vi "HW_Setup.vi"(0 "VISA resource name in":refnum<visa-resource-name>="ASRL3::INSTR", 1 "Traget FPS":i32=80, 2 "Close port? (T)":bool=TRUE, 3 "error in":errorcluster) -> (5 "Version information":string, 6 "VISA resource name out":refnum<visa-resource-name>="ASRL3::INSTR", 7 "Data flow controls":T1, 8 "Instrument OK?":bool=TRUE, 9 "error out":errorcluster)   [LabVIEW 2016]
panel:
  out "FPS status":i32=80
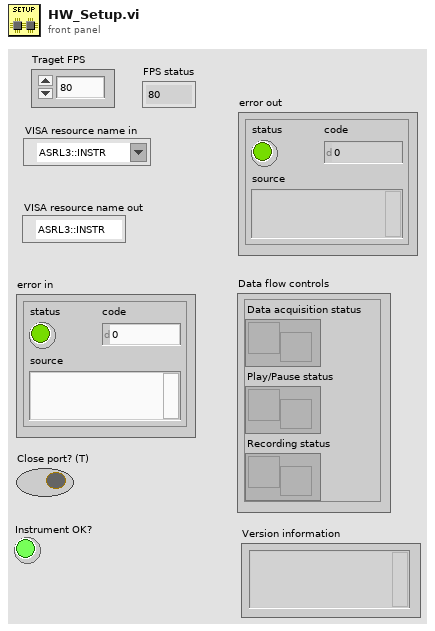
[diagram p1: front panel]
types:
  T1 = cluster{"Data acquisition status":refnum<notifier>, "Play/Pause status":refnum<notifier>, "Recording status":refnum<notifier>}
  T2 = cluster{"notifier out":refnum<notifier>, "notifier out":refnum<notifier>, "notifier out":refnum<notifier>}
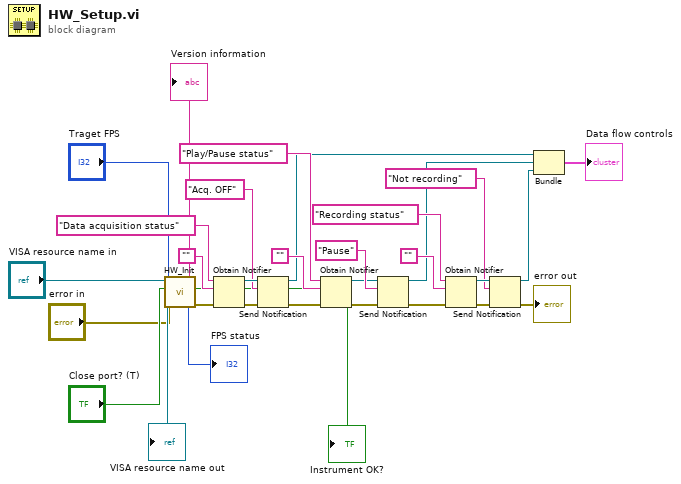
[diagram p0: block diagram]
diagram:
  n1 = call "HW_Init.vi"("error in"="error in", "Traget FPS"="Traget FPS", "Close port? (T)"="Close port? (T)", "VISA resource name"="VISA resource name in") -> ("error out"=w29:errorcluster, "Instrument OK?"=→"Instrument OK?":bool, "VISA resource name out"=→"VISA resource name out":refnum<visa-resource-name>, "FPS status"=→"FPS status":i32, "Version information"=→"Version information":string)  [unwired: 1 out]
  n2 = Obtain Notifier(name (unnamed)="Data acquisition status", notification data type="", error in (no error)=w29) -> (notifier out=w26:refnum<notifier>, error out=w24:errorcluster)  [unwired: 1 in, 1 out]
  n3 = Send Notification(notification="Acq. OFF", notifier=w26, error in (no error)=w24) -> (notifier out=w10:refnum<notifier>, error out=w18:errorcluster)
  n4 = Obtain Notifier(name (unnamed)="Play/Pause status", notification data type="", error in (no error)=w18) -> (notifier out=w21:refnum<notifier>, error out=w23:errorcluster)  [unwired: 1 in, 1 out]
  n5 = Send Notification(notification="Pause", notifier=w21, error in (no error)=w23) -> (notifier out=w9:refnum<notifier>, error out=w12:errorcluster)
  n6 = Obtain Notifier(name (unnamed)="Recording status", notification data type="", error in (no error)=w12) -> (notifier out=w15:refnum<notifier>, error out=w13:errorcluster)  [unwired: 1 in, 1 out]
  n7 = Send Notification(notification="Not recording", notifier=w15, error in (no error)=w13) -> (notifier out=w8:refnum<notifier>, error out=→"error out":errorcluster)
  n8 = Bundle("notifier out"=w10, "notifier out"=w9, "notifier out"=w8) -> (→"Data flow controls":T2)  [unwired: 1 in]
